vi "Log If Error.vi"(4 "Event Time":timestamp, 6 "Include Warnings(F)":bool, 7 "Event Level (Error)":T1=enum."Error", 8 "Error In":errorcluster, 9 "Clear After Logging?(F)":bool, 11 "SourceID":string) -> (0 "error out":errorcluster)   [LabVIEW 2018, in "MVA Framework.lvlib" / "Singleton Event Log.lvlib"]
uses:
  Singleton Event Log.lvlib
  LoggerReference/LoggerReference.lvclass
  Types/Log Level.ctl
  Composed Log.lvlib
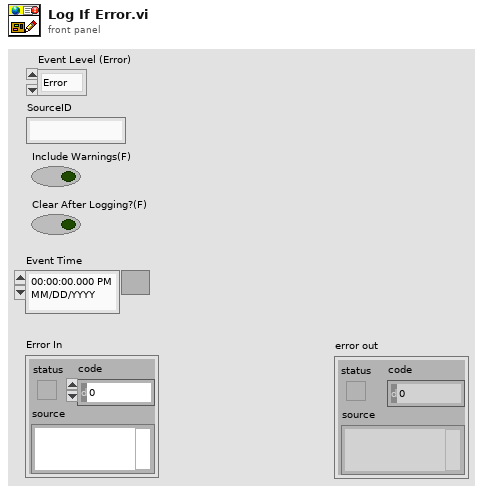
[diagram p1: front panel]
types:
  T1 = typedef "MVA Framework.lvlib/Composed Log.lvlib/Log Level.ctl" = enum16{"Debug", "Info", "Warning", "Error", "Critical"}
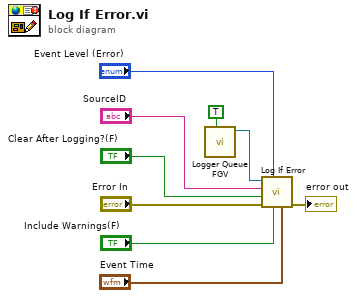
[diagram p0: block diagram]
diagram:
  n1 = call "Logger Queue FGV.vi"("Read?"=TRUE) -> ("LogReference Instance Out"=w8:refnum<class "LoggerReference.lvclass">)  [unwired: 10 in]
  n2 = call "Log If Error.vi"("Event Time"="Event Time", "Include Warnings(F)"="Include Warnings(F)", "Event Level (Error)"="Event Level (Error)", "Error In"="Error In", "Clear After Logging?(F)"="Clear After Logging?(F)", "SourceID"="SourceID", "Log Instance"=w8) -> ("error out"=→"error out":errorcluster)  [unwired: 3 in, 1 out]
